vi "Write instances allowed.vi"(8 "error in":errorcluster, 10 "instances allowed":i32, 11 "DecideProjectFeatures in":refnum<class "DCAFConfigurablePluginDecideFeatures.lvclass">) -> (0 "error out":errorcluster, 3 "DecideProjectFeatures out":refnum<class "DCAFConfigurablePluginDecideFeatures.lvclass">)   [LabVIEW 2013, in "DCAFConfigurablePluginDecideFeatures.lvclass"]
uses:
  DCAFConfigurablePluginDecideFeatures.lvclass
  DCAFConfigurablePluginDecideFeatures.lvclass/DCAFConfigurablePluginDecideFeatures.ctl
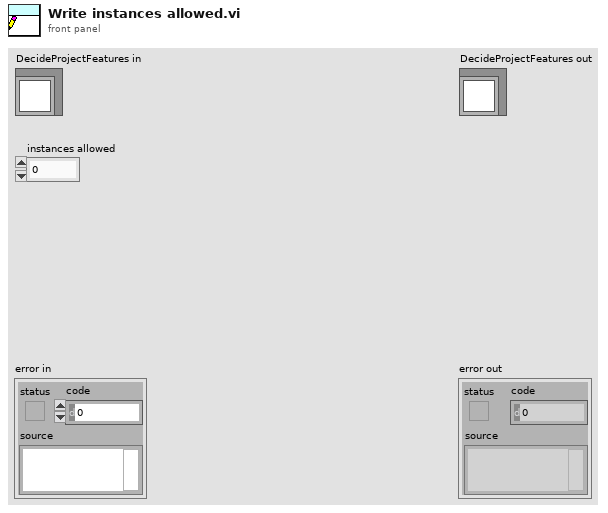
[diagram p1: front panel]
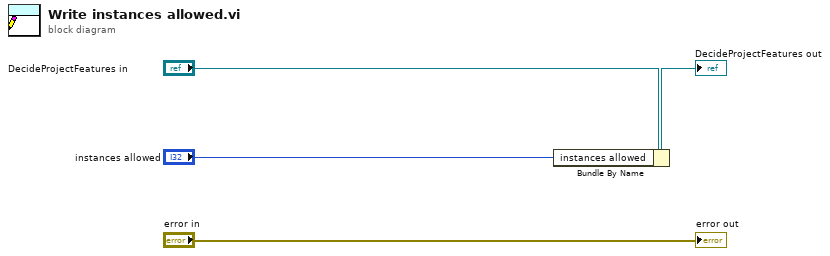
[diagram p0: block diagram]
diagram:
  n1 = Bundle By Name(cluster="DecideProjectFeatures in", "instances allowed"="instances allowed") -> (→"DecideProjectFeatures out":refnum<class "DCAFConfigurablePluginDecideFeatures.lvclass">)
  "error out" <- "error in"
